vi "Update Target Frequency.vi"(7 "New Target Frequency":dbl=100.0, 8 "error in (no error)":errorcluster, 11 "TimerDRV in":refnum<class "TimerDRV.lvclass">) -> (0 "error out":errorcluster, 3 "TimerDRV out":refnum<class "TimerDRV.lvclass">)   [LabVIEW 2019, in "TimingDRV Engine.lvlib" / "TimerDRV.lvclass"]
uses:
  TimerDRV.lvclass
  TimerDRV.lvclass/TimerDRV.ctl
  <vilib>/Utility/error.llb/Error Cluster From Error Code.vi
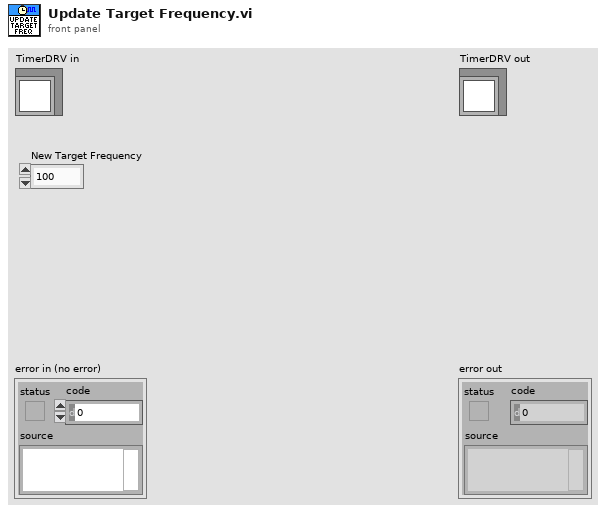
[diagram p1: front panel]
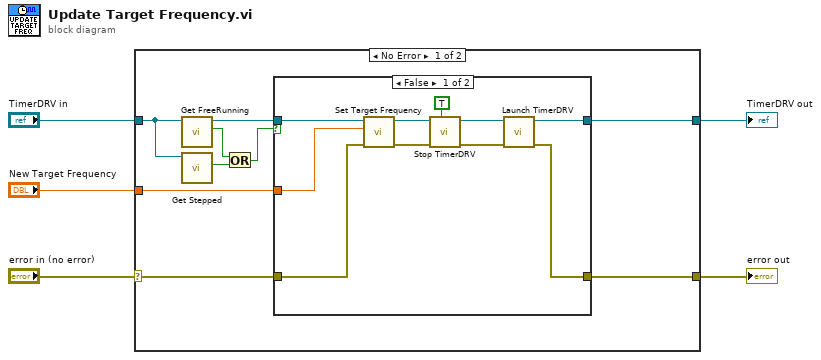
[diagram p0: block diagram]
diagram:
  n1 = case shown="No Error" "error in (no error)" {
    selector: "error in (no error)" -> [w11 w28]
    tunnel: [w12 w28] -> w4
    tunnel: [w13 w27] -> w2
    tunnel: "TimerDRV in" -> [w9 w27]
    tunnel: "New Target Frequency" -> [w14 _]
    frame No Error {
      n2 = call "Get FreeRunning.vi"("TimerDRV in"=w9) -> ("FreeRunning"=w7:bool, "TimerDRV out"=w10:refnum<class "TimerDRV.lvclass">)  [unwired: 9 in]
      n3 = call "Get Stepped.vi"("TimerDRV in"=w9) -> ("Stepped"=w8:bool)  [unwired: 9 in, 1 out]
      n4 = Or(x=w7, y=w8) -> (x .or. y?=w6:bool)
      n5 = case shown="False" w6 {
        tunnel: w14 -> [w24 _]
        tunnel: [w20 w25] -> w13
        tunnel: [w19 w26] -> w12
        tunnel: w11 -> [w17 w26]
        tunnel: w10 -> [w15 w25]
        frame False {
          n6 = call "Set Target Frequency.vi"("Error In"=w17, "Target Frequency"=w24, "TimerDRV in"=w15) -> ("Error Out"=w16:errorcluster, "TimerDRV out"=w23:refnum<class "TimerDRV.lvclass">)  [unwired: 7 in]
          n7 = call "Stop TimerDRV.vi"("Keep Time Source?"=TRUE, "error in (no error)"=w16, "TimerDRV in"=w23) -> ("error out"=w21:errorcluster, "TimerDRV out"=w22:refnum<class "TimerDRV.lvclass">)  [unwired: 7 in]
          n8 = call "Launch TimerDRV.vi"("error in (no error)"=w21, "TimerDRV in"=w22) -> ("error out"=w19:errorcluster, "TimerDRV out"=w20:refnum<class "TimerDRV.lvclass">)  [unwired: 8 in]
        }
        frame True {
        }
      }
    }
    frame Error {
    }
  }
  "error out" <- w4
  "TimerDRV out" <- w2
